vi "sub 3.vi"(8 "error in (no error)":errorcluster) -> (0 "error out":errorcluster, 3 "File Refnum Out":refnum<file>)   [LabVIEW 2015]
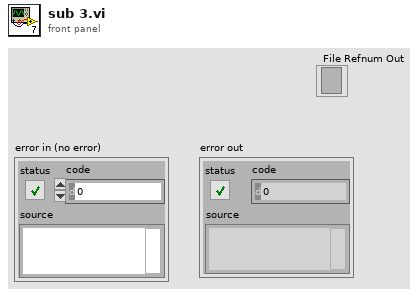
[diagram p1: front panel]
types:
  T1 = enum16{"open", "replace", "create", "open or create", "replace or create", "replace or create with confirmation"}
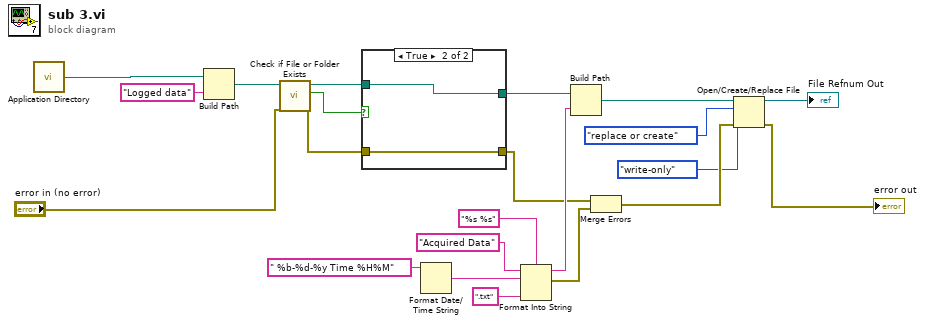
[diagram p0: block diagram]
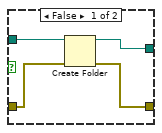
[diagram p2: hidden frame]
diagram:
  n1 = call <vilib>:"Application Directory.vi"() -> ("Application Directory"=w1:path)
  n2 = Build Path(base path=w1, name or relative path="Logged data") -> (appended path=w7:path)
  n3 = call <vilib>:"Check if File or Folder Exists.vi"("error in (no error)"="error in (no error)", "path"=w7) -> ("error out"=w3:errorcluster, "file or folder exists?"=w4:bool, "dup path"=w5:path)  [unwired: 7 in]
  n4 = case shown="True" w4 {
    tunnel: w3 -> [w24 w27]
    tunnel: w5 -> [w26 w28]
    tunnel: [w25 w28] -> w20
    tunnel: [w23 w27] -> w15
    frame False {
      n5 = Create Folder(path (use dialog)=w26, error in=w24) -> (created path=w25:path, error out=w23:errorcluster)  [unwired: 1 in, 1 out]
    }
    frame True {
    }
  }
  n6 = Format Date/Time String(time format string (%c)=" %b-%d-%y Time %H%M") -> (date/time string=w17:string)  [unwired: 2 in]
  n7 = Format Into String(format string="%s %s", initial string="Acquired Data", w17, ".txt" ("input 2")) -> (resulting string=w19:string, error out=w14:errorcluster)  [unwired: 1 in]
  n8 = Build Path(base path=w20, name or relative path=w19) -> (appended path=w13:path)
  n9 = Merge Errors(w15, w14) -> (w12:errorcluster)
  n10 = Open/Create/Replace File(file path (use dialog)=w13, error in=w12, operation (0:open)=T1."replace or create", access (0:read/write)=enum16{"read/write", "read-only", "write-only"}."write-only") -> (refnum out=→"File Refnum Out":refnum<file>, error out=→"error out":errorcluster)  [unwired: 2 in, 1 out]
